vi "Test Suite Result Error Count.vi"(8 "error in (no error)":errorcluster, 11 "Test Suite Result Test In":refnum<class "Test Suite Result Test.lvclass">) -> (0 "error out":errorcluster, 3 "Test Suite Result Test Out":refnum<class "Test Suite Result Test.lvclass">)   [LabVIEW 2020, in "LUnit Tests.lvlib" / "Test Suite Result Test.lvclass"]
uses:
  Test Suite Result Test.lvclass
  Test Suite Result Test.lvclass/Test Suite Result Test.ctl
  Test Dummys/Test Test Case/Test Test Case.lvclass
  source/Framework/Result Types/Suite Results/Test Suite Result.lvlib
  2dc45940-7be3-4481-8ea7-f550c62a0390.vi
  C:/Git/astemes-lunit/source/Framework/Test Case/LUnit Test Case.lvclass
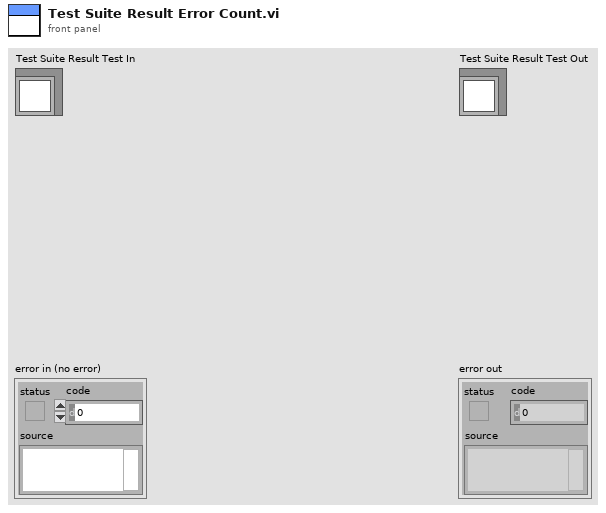
[diagram p1: front panel]
types:
  T1 = typedef "Test Suite Result.lvlib/Test Suite Result.ctl" = cluster{"Test Suite ID":string, "Name":string, "Hostname":string, "Status":T2, "Execution time":dbl, "Start Time":timestamp, "Case Results":T3[]}
  T2 = typedef "Assertion Result.lvlib/Status.ctl" = enum16{"Pass", "Fail", "Error", "Skipped", "Setup Error", "Broken", "Teardown Error"}
  T3 = typedef "Test Case Result.lvlib/Test Case Result.ctl" = map{string, T4}
  T4 = typedef "Method Result.lvlib/Method Result.ctl" = cluster{"Test Case":string, "Test Method Name":string, "Status":T2, "Assertion Results":T5[], "Execution time":dbl, "Result String":string}
  T5 = typedef "Assertion Result.lvlib/Assertion Result.ctl" = cluster{"Status":T2, "Message":string, "Description":string, "Assertion Type":T6}
  T6 = typedef "Assertion Result.lvlib/Assertion Type.ctl" = enum16{"None", "Pass", "Fail", "Skip", "Pass if Equal", "Fail if Equal", "Pass if Error", "Fail if Error", "Pass if", "Fail if"}
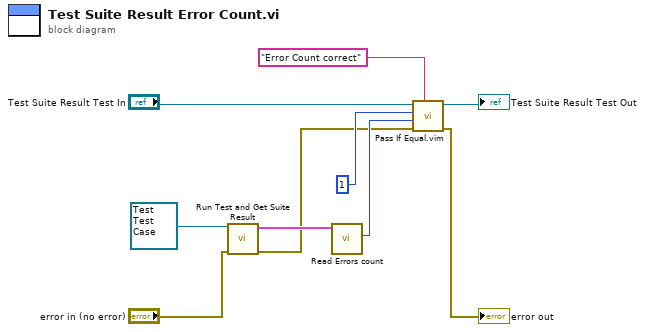
[diagram p0: block diagram]
diagram:
  n1 = call "Run Test and Get Suite Result.vi"("error in (no error)"="error in (no error)", "Test Test Case in"=refnum<class "Test Test Case.lvclass"> refnum ("Test Test Case.lvclass")) -> ("error out"=w3:errorcluster, "Test Suite Result out"=w4:T1)  [unwired: 8 in]
  n2 = call "Read Errors count.vi"("Test Suite Result In"=w4) -> ("Errors count"=w9:i32)  [unwired: 8 in, 2 out]
  n3 = call "Pass If Equal.vim"("Description"="Error Count correct", "error in (no error)"=w3, "Actual"=w9, "Expected"=1 ("x"), "LUnit Test Case In"="Test Suite Result Test In") -> ("error out"=→"error out":errorcluster, "LUnit Test Case Out"=→"Test Suite Result Test Out":refnum<class "Test Suite Result Test.lvclass">)  [unwired: 5 in]
